vi "Register 0 Write.vi"(0 "instrument handle in":refnum<k15>, 1 "Bus Number":i32, 5 "Slave Address":T2=12 format="%02x", 7 "Register Data":T1 format="%02x", 11 "error in (no error)":errorcluster) -> (4 "instrument handle out":refnum<k15>, 15 "error out":errorcluster)   [LabVIEW 2018, in "MIPI RFFE API.lvlib"]
uses:
  MIPI RFFE API.lvlib
  Slave Address.ctl
  Register Data.ctl
  Reg0Write/RFFE Reg0Write Command.lvclass
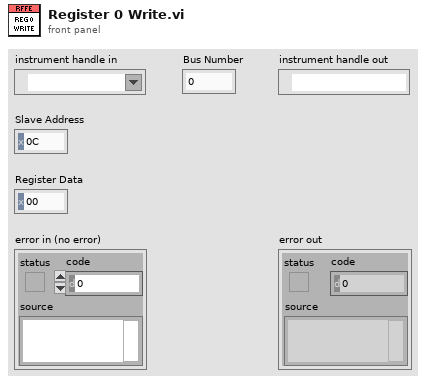
[diagram p1: front panel]
types:
  T1 = typedef "MIPI RFFE API.lvlib/Register Data.ctl" = u8
  T2 = typedef "MIPI RFFE API.lvlib/Slave Address.ctl" = u8
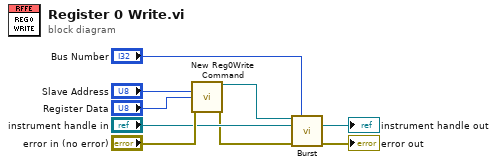
[diagram p0: block diagram]
diagram:
  n1 = call "New Reg0Write Command.vi"("Slave Address"="Slave Address", "Register Data"="Register Data", "error in (no error)"="error in (no error)") -> ("RFFE Reg0Write Command out"=w2:refnum<class "RFFE Reg0Write Command.lvclass">, "error out"=w1:errorcluster)  [unwired: 11 in]
  n2 = call-dynamic "Burst.vi"("RFFE Command in"=w2, "Bus Number"="Bus Number", "instrument handle in"="instrument handle in", "error in (no error)"=w1) -> ("instrument handle out"=→"instrument handle out":refnum<k15>, "error out"=→"error out":errorcluster)  [unwired: 9 in, 1 out]
